vi "DQMH_Group Modules.vi"(0 "Module 6":T1, 4 "Module 5":T1, 6 "Module 4":T1, 8 "error in (no error)":errorcluster, 9 "Module 3":T1, 10 "Module 2":T1, 11 "Module 1":T1) -> (1 "error out":errorcluster, 3 "Modules":T1)   [LabVIEW 2025]
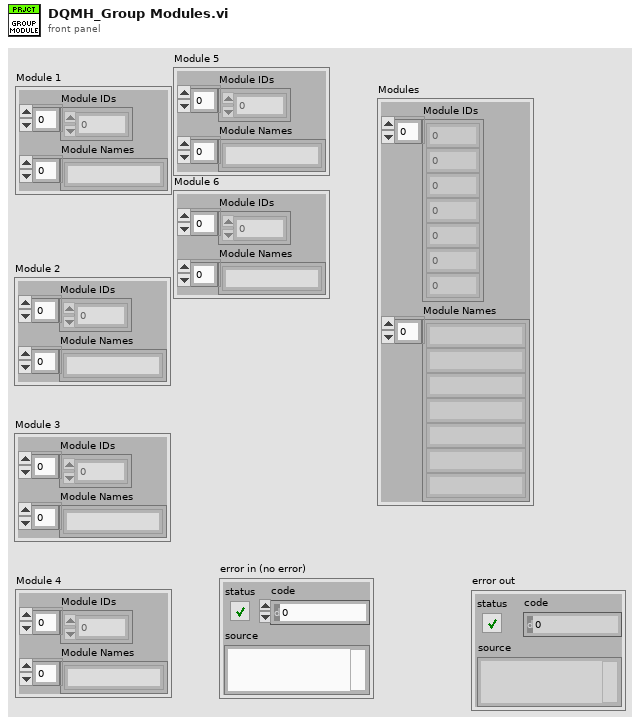
[diagram p1: front panel]
types:
  T1 = cluster{"Module IDs":i32[], "Module Names":string[]}
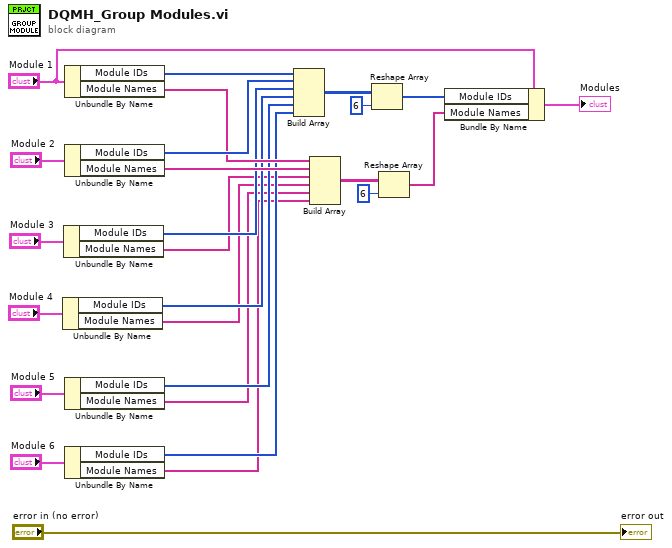
[diagram p0: block diagram]
diagram:
  n1 = Unbundle By Name("Module 4") -> ("Module IDs"=w8:i32[], "Module Names"=w4:string[])
  n2 = Unbundle By Name("Module 3") -> ("Module IDs"=w9:i32[], "Module Names"=w5:string[])
  n3 = Unbundle By Name("Module 1") -> ("Module IDs"=w25:i32[], "Module Names"=w23:string[])
  n4 = Unbundle By Name("Module 2") -> ("Module IDs"=w24:i32[], "Module Names"=w22:string[])
  n5 = Unbundle By Name("Module 5") -> ("Module IDs"=w7:i32[], "Module Names"=w3:string[])
  n6 = Unbundle By Name("Module 6") -> ("Module IDs"=w6:i32[], "Module Names"=w2:string[])
  n7 = Build Array(w25, w24, w9, w8, w7, w6) -> (w20:i32[][])
  n8 = Build Array(w23, w22, w5, w4, w3, w2) -> (w17:string[][])
  n9 = Reshape Array(w20, 6 ("dimension size")) -> (w19:i32[])
  n10 = Reshape Array(w17, 6 ("dimension size")) -> (w16:string[])
  n11 = Bundle By Name(cluster="Module 1", "Module IDs"=w19, "Module Names"=w16) -> (→"Modules":T1)
  "error out" <- "error in (no error)"
